vi "倒计时.vi"() -> ()   [LabVIEW 2017]
panel:
  in  "停止":bool
  out "倒计时":string
  out "倒计时器":bool
  in  "开始倒计时":bool
  in  "定时时间选择":enum16{"20秒", "10秒", "6秒"}(ring)
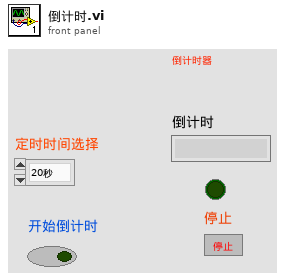
[diagram p1: front panel]
types:
  T1 = enum8{"Enabled", "Disabled", "Disabled and Grayed Out"}
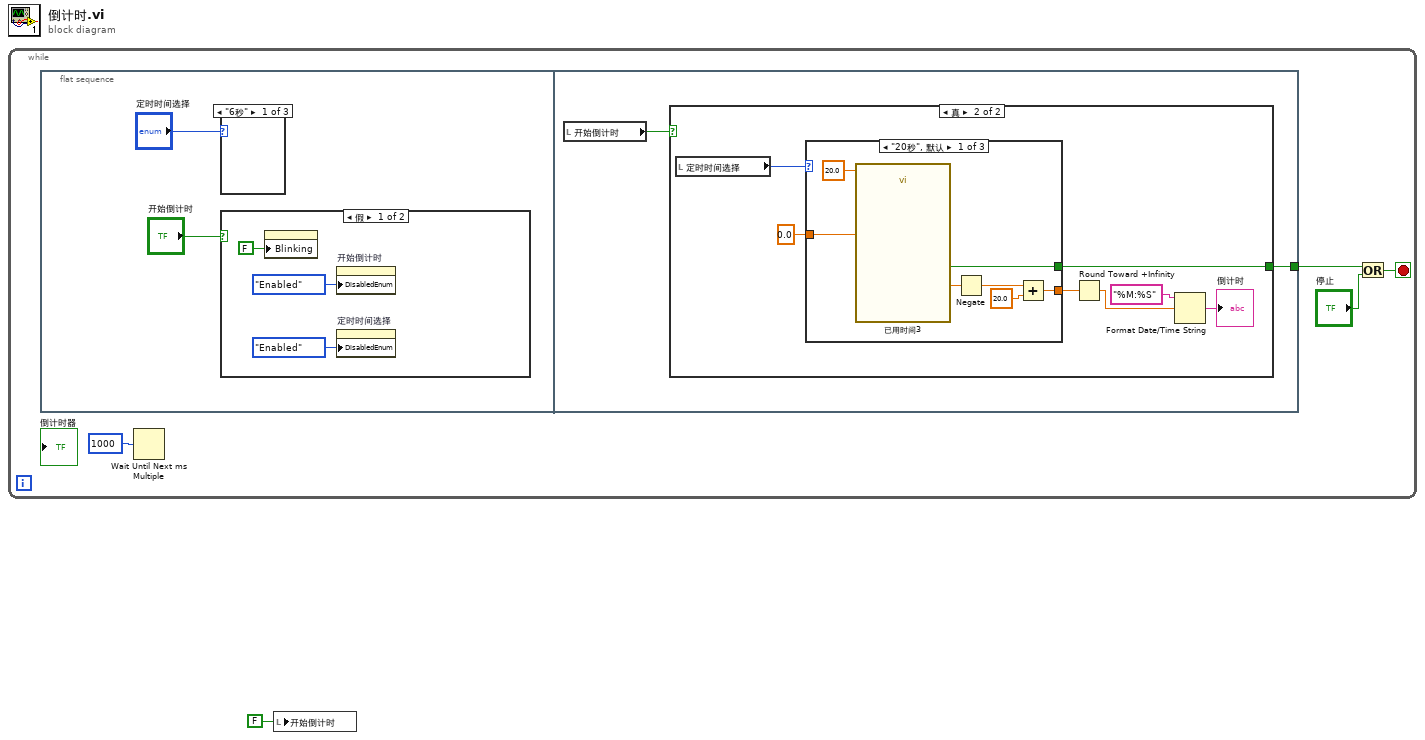
[diagram p0: block diagram]
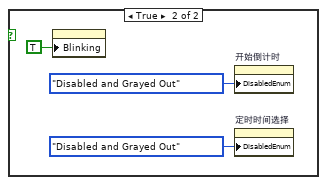
[diagram p2: hidden frame]
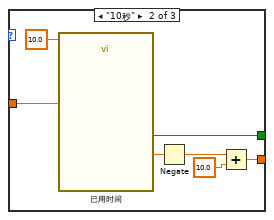
[diagram p6: hidden frame]
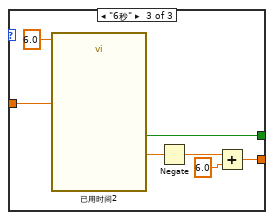
[diagram p7: hidden frame]
diagram:
  n1 = while {
    stop <- w4 stop-if-true
    n2 = flat-sequence {
      tunnel: [w14] -> w2
      frame #0 {
        n3 = case shown="\"6秒\"" "定时时间选择" {
          frame "6秒" {
          }
          frame "10秒" {
          }
          frame "20秒" {
          }
        }
        n4 = case shown="假" "开始倒计时" {
          frame False {
            n5 = property on="倒计时器" class="Bool (严格)"("Blinking"=FALSE ("闪烁")) -> ()  [unwired: 2 in, 2 out]
            n6 = property on="开始倒计时" class="Bool (严格)"("DisabledEnum"=T1."Enabled" ("禁用")) -> ()  [unwired: 2 in, 2 out]
            n7 = property on="定时时间选择" class="Enum (严格)"("DisabledEnum"=T1."Enabled" ("禁用")) -> ()  [unwired: 2 in, 2 out]
          }
          frame True {
            n8 = property on="倒计时器" class="Bool (严格)"("Blinking"=TRUE ("闪烁")) -> ()  [unwired: 2 in, 2 out]
            n9 = property on="开始倒计时" class="Bool (严格)"("DisabledEnum"=T1."Disabled and Grayed Out" ("禁用")) -> ()  [unwired: 2 in, 2 out]
            n10 = property on="定时时间选择" class="Enum (严格)"("DisabledEnum"=T1."Disabled and Grayed Out" ("禁用")) -> ()  [unwired: 2 in, 2 out]
          }
        }
      }
      frame #1 {
        n11 = local read "开始倒计时"() -> (w15:bool)
        n12 = case shown="真" w15 {
          tunnel: [_ w16] -> w14
          frame False {
          }
          frame True {
            n13 = local read "定时时间选择"() -> (w17:enum16{"20秒", "10秒", "6秒"})
            n14 = case shown="\"20秒\", 默认" w17 {
              tunnel: 0.0 ("Set Start Time (s)") -> [w28 w35 w42]
              tunnel: [w24 w31 w39] -> w21
              tunnel: [w23 w30 w37] -> w16
              frame "20秒", Default {
                n15 = call "已用时间3"("Time Target (s)"=20.0, "Set Start Time (s)"=w28) -> ("Elapsed Time (s)"=w27:dbl, "Time has Elapsed"=w23:bool)  [unwired: 10 in, 6 out]
                n16 = Negate(x=w27) -> (-x=w26:dbl)
                n17 = Add(x=w26, y=20.0) -> (x+y=w24:dbl)
              }
              frame "10秒" {
                n18 = call "已用时间"("Time Target (s)"=10.0, "Set Start Time (s)"=w35) -> ("Elapsed Time (s)"=w34:dbl, "Time has Elapsed"=w30:bool)  [unwired: 10 in, 6 out]
                n19 = Negate(x=w34) -> (-x=w33:dbl)
                n20 = Add(x=w33, y=10.0) -> (x+y=w31:dbl)
              }
              frame "6秒" {
                n21 = call "已用时间2"("Time Target (s)"=6.0, "Set Start Time (s)"=w42) -> ("Elapsed Time (s)"=w41:dbl, "Time has Elapsed"=w37:bool)  [unwired: 10 in, 6 out]
                n22 = Negate(x=w41) -> (-x=w40:dbl)
                n23 = Add(x=w40, y=6.0) -> (x+y=w39:dbl)
              }
            }
            n24 = Round Toward +Infinity(x=w21) -> (ceil(x): smallest int >= x=w20:dbl)
            n25 = Format Date/Time String(time format string (%c)="%M:%S" ("时间格式字符串(%c)"), seconds (now)=w20) -> (date/time string=→"倒计时":string)  [unwired: 1 in]
          }
        }
      }
    }
    n26 = Wait Until Next ms Multiple(millisecond multiple=u32 1000 ("毫秒倍数")) -> ()  [unwired: 1 out]
    n27 = Or(x=w2, y="停止") -> (x .or. y?=w4:bool)
  }
  n28 = local write "开始倒计时"(FALSE ("开始倒计时")) -> ()
